vi "Read Children Chromosomes.vi"(8 "error in (no error)":errorcluster, 11 "IPopulation in":refnum<class "IPopulation.lvclass">) -> (0 "error out":errorcluster, 2 "Children Chromosomes":refnum<data-value>, 3 "IPopulation out":refnum<class "IPopulation.lvclass">)   [LabVIEW 2016, in "IPopulation.lvclass"]
uses:
  IPopulation.lvclass
  IChromosome/IChromosome.lvclass
  IPopulation.lvclass/IPopulation.ctl
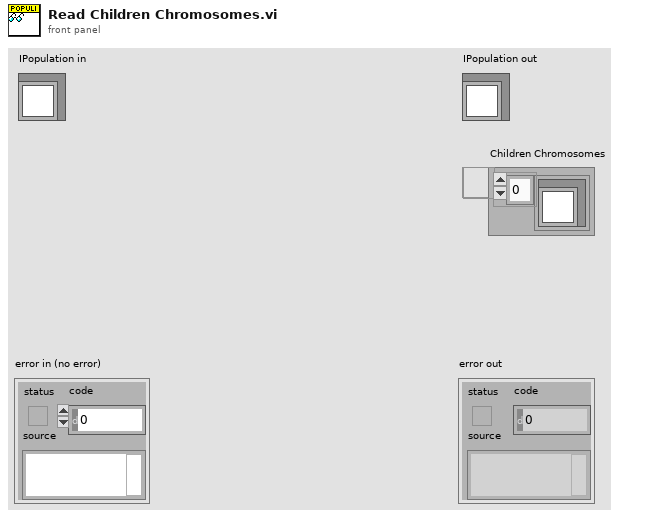
[diagram p1: front panel]
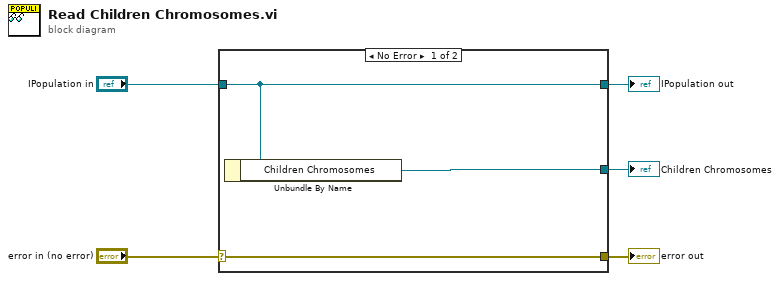
[diagram p0: block diagram]
diagram:
  n1 = case shown="No Error" "error in (no error)" {
    selector: "error in (no error)" -> [w8 w9]
    tunnel: [w8 w9] -> w4
    tunnel: [w7 w10] -> w2
    tunnel: "IPopulation in" -> [w7 w10]
    tunnel: [w6 _] -> w1
    frame No Error {
      n2 = Unbundle By Name(w7) -> ("Children Chromosomes"=w6:refnum<data-value>)
    }
    frame Error {
    }
  }
  "error out" <- w4
  "IPopulation out" <- w2
  "Children Chromosomes" <- w1
